vi "Freio_Histerese.vi"(2 "error in Fonte_Freio_Handle":errorcluster, 3 "VISA in Fonte_Freio_Handle":refnum<visa-resource-name>="GPIB::6::INSTR") -> (0 "error out Fonte_Freio_Handle":errorcluster, 1 "VISA out Fonte_Freio_Handle":refnum<visa-resource-name>)   [LabVIEW 2025]
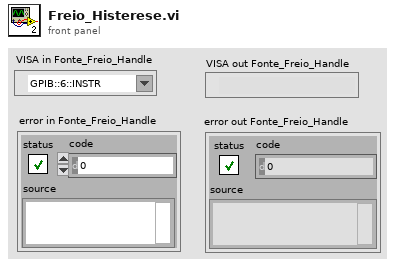
[diagram p1: front panel]
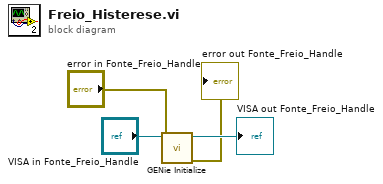
[diagram p0: block diagram]
diagram:
  n1 = call <instrlib>:"GENie Initialize.vi"("error in (no error)"="error in Fonte_Freio_Handle", "VISA name"="VISA in Fonte_Freio_Handle") -> ("error out"=→"error out Fonte_Freio_Handle":errorcluster, "VISA out"=→"VISA out Fonte_Freio_Handle":refnum<visa-resource-name>)  [unwired: 8 in]
